vi "g_Pos_Determine.vi"() -> ()   [LabVIEW 2015, in "ExcuseNotesHandler.lvclass"]
uses:
  ExcuseNotesHandler.lvclass
panel:
  in  "Pos_Date":i32=3
  in  "Pos_Reason":i32=5
  in  "Pos_Time":i32=4
  in  "Pos_Determine":i32=6
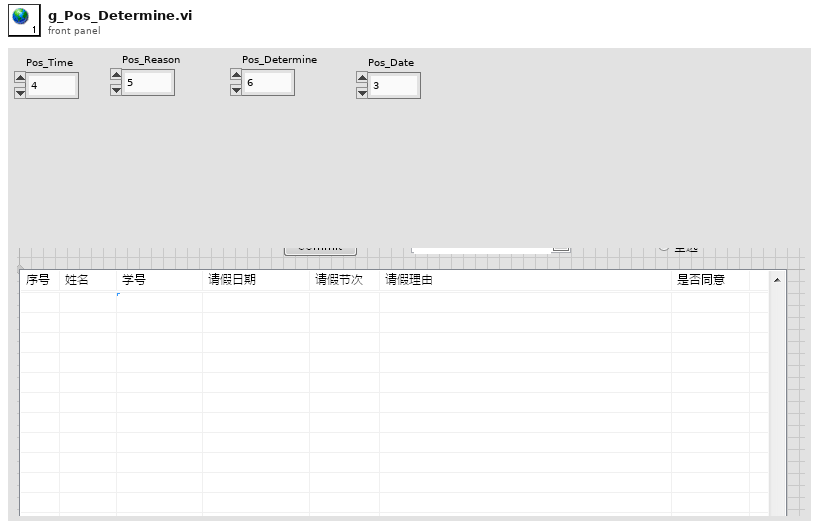
[diagram p1: front panel]
diagram:
